vi "ModbusManual.vi"() -> ()   [LabVIEW 2018, in "ScratchpadLibrary.lvlib"]
uses:
  ScratchpadLibrary.lvlib
  <vilib>/Platform/TimedLoop/XDataNode/timing_clust.ctl
  <vilib>/Platform/TimedLoop/XDataNode/nitl_modes.ctl
  <vilib>/Platform/TimedLoop/XDataNode/wakeup.ctl
  <vilib>/Modbus/master/Create Master Instance (Serial).vi
  <vilib>/platform/TimedLoop/XDataNode/XDataNode.xnode
  <vilib>/Modbus/master/Modbus Master.lvclass
  <vilib>/Platform/TimedLoop/XDataNode/XDNodeRunTimeDep.lvlib
panel:
  out "(hi.lo)":u32 format="%x"
  out "*(type *) &x":sgl
  out "element":u16
  out "error out":errorcluster
  in  "Stop":bool
  in  "Frequency":dbl(slide) scale=0.1..10.0
  out "Interval":i64
  out "Counter":i32
  out "Time (ms)":u32
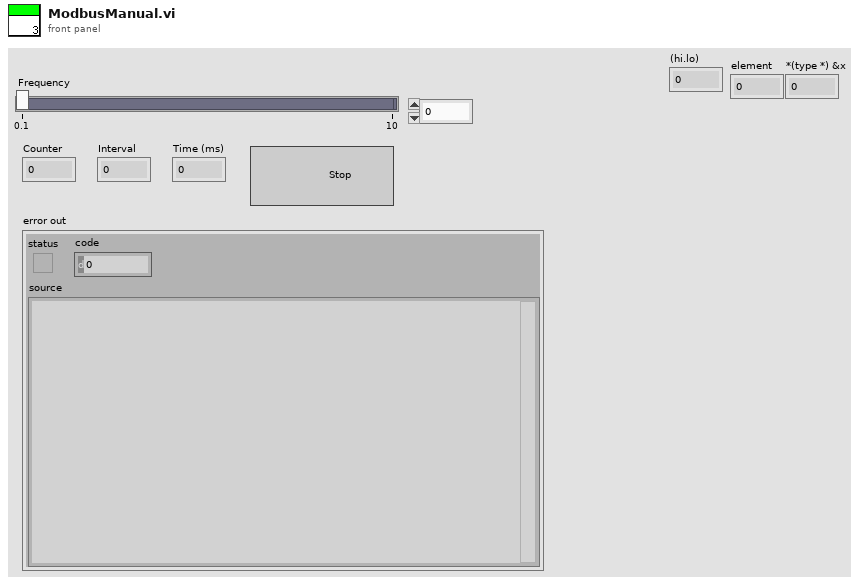
[diagram p1: front panel]
types:
  T1 = typedef "XDNodeRunTimeDep.lvlib/timing_clust.ctl" = cluster{"Expected End [f-1]":u64, "Actual End [f-1]":u64, "Finished Late? [f-1]":bool, "Expected End [i-1]":u64, "Actual End [i-1]":u64, "Finished Late? [i-1]":bool, "Expected Start [i]":u64, "Actual Start [i]":u64, "Expected Start [f]":u64, "Actual Start [f]":u64, "Source Name":string, "Structure Name":string, "Period":i64, "Deadline":i64, "Offset":i64, "Start":i64, "Priority":i32, "Timeout":i32, "Mode":T2, "Wakeup Reason":T3, "Error":errorcluster, "Source Type":string, "Secondary Source Type":string, "Global End Time":u64, "Global Start Time":u64, "Frame Duration":u64, "Iteration Duration":u64, "Assigned CPU":i32, "I/O Scan Engine Mode":u32}
  T2 = typedef "XDNodeRunTimeDep.lvlib/nitl_modes.ctl" = enum32{"No Change", "Process missed periods, maintain original phase", "Discard missed periods, maintain original phase", "Process missed periods, ignore original phase", "Discard missed periods, ignore original phase"}
  T3 = typedef "XDNodeRunTimeDep.lvlib/wakeup.ctl" = enum32{"Normal", "Aborted", "Asynchronous wakeup", "Timing source error", "Timed loop error", "Timeout"}
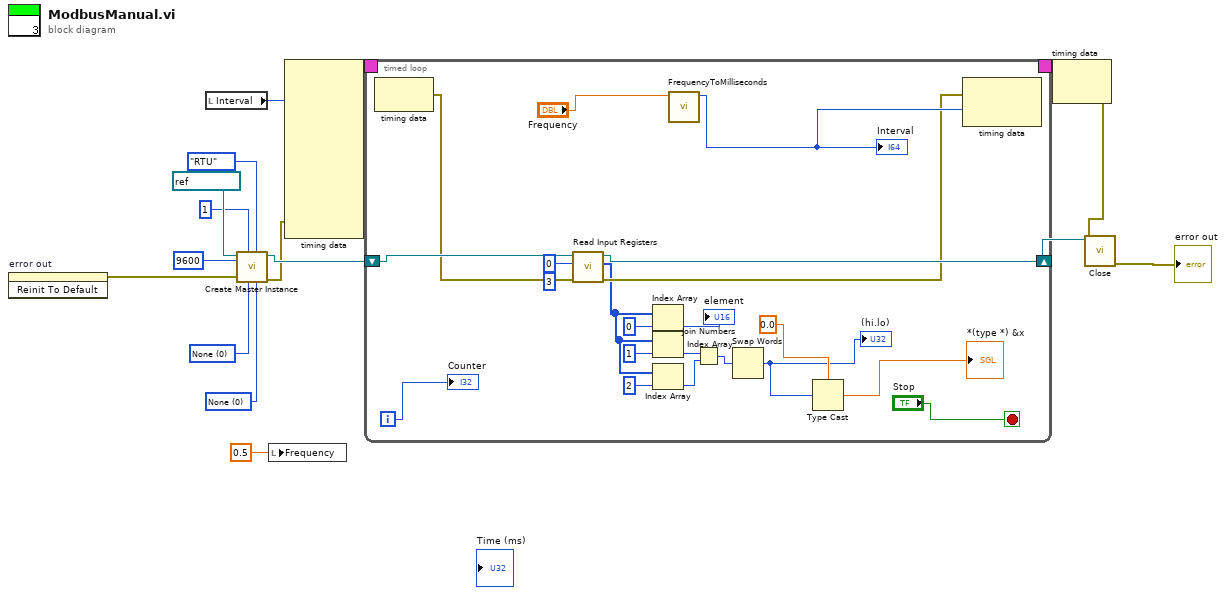
[diagram p0: block diagram]
diagram:
  w5 = u16 0 items=["None", "XON/XOFF", "RTS/CTS", "XON/XOFF & RTS/CTS", "DTR/DSR", "XON/XOFF & DTR/DSR"] ("flow control (None)")
  w6 = u16 0 items=["None", "Odd", "Even"] ("parity (Even)")
  n1 = invoke on="error out" class="Clust (strict)" method="Reinit To Default"() -> (error out=w2:errorcluster)  [unwired: 3 in, 2 out]
  n2 = local read "Interval"() -> (w14:i64)
  n3 = call-poly <vilib>:"Create Master Instance.vi"("flow control (None)"=w5, "serial type"=enum16{"RTU", "ASCII"}."RTU", "parity (Even)"=w6, "unit ID"=u8 1, "error in (no error)"=w2, "baud rate (9600)"=u32 9600, "VISA resource name"=refnum<visa-resource-name> "COM11") -> ("error out"=w9:errorcluster, "serial master instance"=w11:refnum<class "Modbus Master.lvclass">)  [unwired: 3 in]
  n4 = local write "Frequency"(0.5 ("Frequency")) -> ()
  n5 = node-c288(w14, w9) -> (w16:T1)  [unwired: 8 in]
  n6 = timed-loop {
    timing: w16 -> [_]
    timing-out: [_] -> w15
    shift-right: [w32] -> w10
    shift-left: w11 -> [w33]
    i -> [w37]
    stop <- "Stop" stop-if-true
    n7 = node-c288() -> (w31:errorcluster)  [unwired: 1 in]
    n8 = call-dynamic "Read Input Registers.vi"("error in (no error)"=w31, "number of input registers"=u16 3, "starting address"=u16 0, "Modbus master in"=w33) -> ("error out"=w30:errorcluster, "register values"=w27:u16[], "Modbus master out"=w32:refnum<class "Modbus Master.lvclass">)  [unwired: 5 in]
    n9 = Index Array(array=w27, index=0) -> (element=→"element":u16)
    n10 = Index Array(array=w27, index=1) -> (element=w20:u16)
    n11 = Index Array(array=w27, index=2) -> (element=w19:u16)
    n12 = call "FrequencyToMilliseconds.vi"("Frequency"="Frequency") -> ("Numeric"=w35:i64)  [unwired: 10 in]
    "Interval" <- w35
    n13 = Join Numbers(hi=w20, lo=w19) -> ((hi.lo)=w18:u32)
    n14 = Swap Words(1:w18) -> (0:w17:u32)
    "(hi.lo)" <- w17
    n15 = Type Cast(type=sgl 0.0, x=w17) -> (*(type *) &x=→"*(type *) &x":sgl)
    n16 = node-c288(w30, w35) -> ()  [unwired: 1 out]
    "Counter" <- w37
  }
  n17 = node-c288(w15) -> (w8:errorcluster)
  n18 = call-dynamic "Close.vi"("error in (no error)"=w8, "Modbus master in"=w10) -> ("error out"=→"error out":errorcluster)  [unwired: 9 in]
